vi "getStepNLoopParams.vi"(0 "Controller in":refnum<class "_Controller.lvclass">, 2 "axis (only applicable to multi-axis applications)":T2, 5 "error in (no error)":errorcluster) -> (14 "Controller out":refnum<class "_Controller.lvclass">, 16 "step_n_params":T1, 19 "error out":errorcluster)   [LabVIEW 2013, in "classes.lvlib" / "_Controller.lvclass"]
doc: "Retreive the Step N Loop paramters for a given axis. For single axis applications, axis need not be specified.\n\nProduced By:\n\n<B>Kod Integrations, LLC</B>\n4835 Marianne Drive\nMount Airy, MD 21771\nhttp://www.kodintegrations.com\nemail: info@kodintegrations.com\nphone: (240) 687-1288"
uses:
  _Controller.lvclass
  common/controls/axis.ctl
  common/controls/step_n_params.ctl
  libraries/common.lvlib
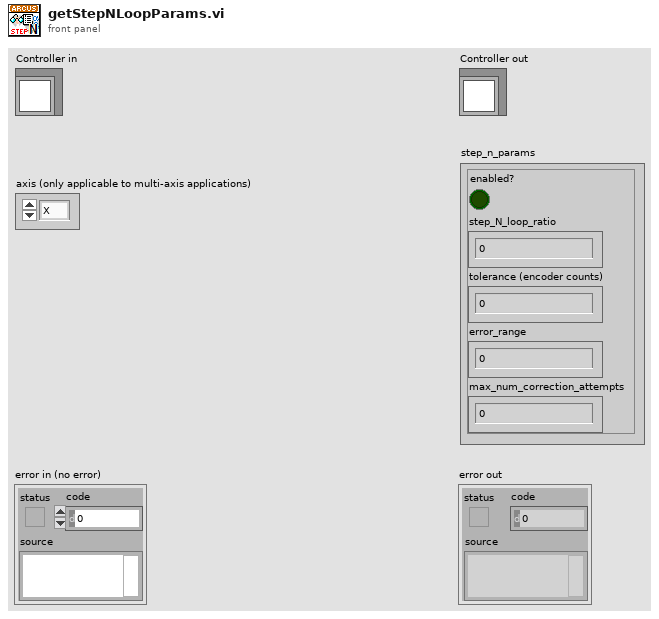
[diagram p1: front panel]
types:
  T1 = typedef "common.lvlib/step_n_params.ctl" = cluster{"step_N_loop_ratio":dbl, "tolerance (encoder counts)":u32, "error_range":i32, "max_num_correction_attempts":i32, "enabled?":bool}
  T2 = typedef "common.lvlib/axis.ctl" = enum16{"X", "Y", "Z", "U"}
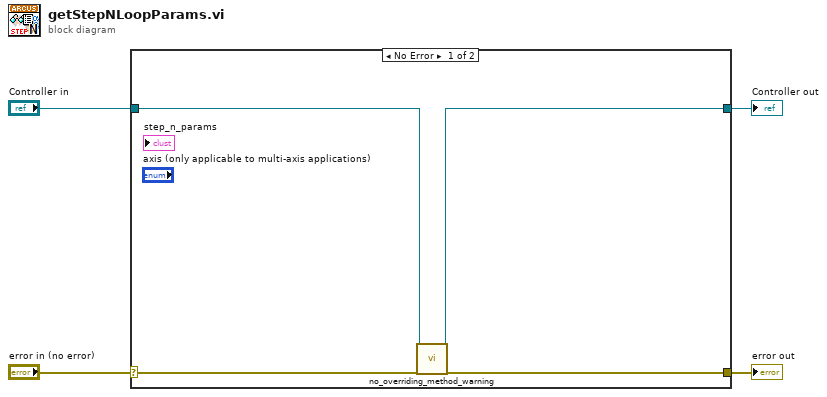
[diagram p0: block diagram]
diagram:
  n1 = case shown="No Error" "error in (no error)" {
    selector: "error in (no error)" -> [w8 w10]
    tunnel: [w7 w10] -> w3
    tunnel: [w5 w9] -> w1
    tunnel: "Controller in" -> [w6 w9]
    frame No Error {
      n2 = call "no_overriding_method_warning.vi"("Controller (in)"=w6, "error in (no error)"=w8) -> ("Controller (out)"=w5:refnum<class "_Controller.lvclass">, "error out"=w7:errorcluster)  [unwired: 15 in, 1 out]
    }
    frame Error {
    }
  }
  "error out" <- w3
  "Controller out" <- w1
